vi "read Rx.vi"(8 "error in (no error)":errorcluster, 9 "length":u16, 10 "protocol_version":i32, 11 "port_num":i32) -> (0 "error out":errorcluster)   [LabVIEW 2018, in "labview.lvlib"]
doc: "WINDECLSPEC void readRx (int port_num, int protocol_version, uint16_t length);"
uses:
  labview.lvlib
  dxl_x86_c.dll
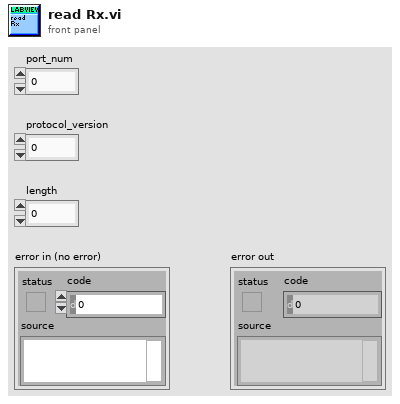
[diagram p1: front panel]
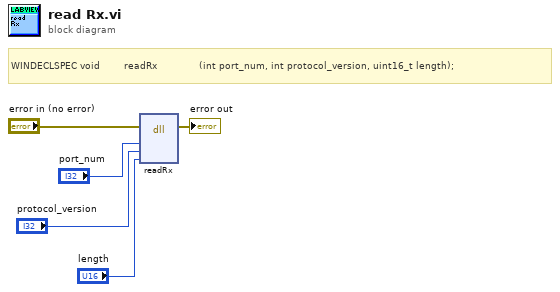
[diagram p0: block diagram]
diagram:
  # "WINDECLSPEC void        readRx              (int port_num, int protocol_version, uint16_t length);"
  n1 = dll-call lib="C:/Users/joaos/OneDrive/Documents/[PhD]/Project Omnidirectional Vehicle/Vanes/LabView_code/joaoandthethreestands/DynamixelSDK-3.7.31/labview/new_compilation/dxl_x86_c.*" fn="readRx"(error in="error in (no error)", "port_num"="port_num", "protocol_version"="protocol_version", "length"="length") -> (error out=→"error out":errorcluster)  [unwired: 6 in, 1 out]
